vi "Call UI Initialize Device.vi"(8 "error in":errorcluster) -> (0 "error out":errorcluster)   [LabVIEW 2019, in "Initialize.lvlib"]
uses:
  Initialize.lvlib
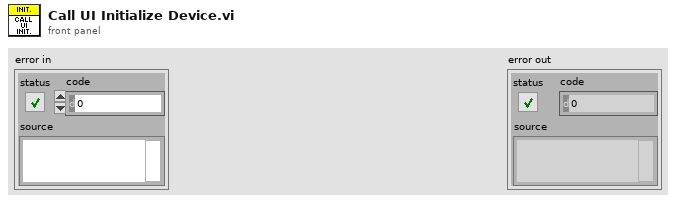
[diagram p1: front panel]
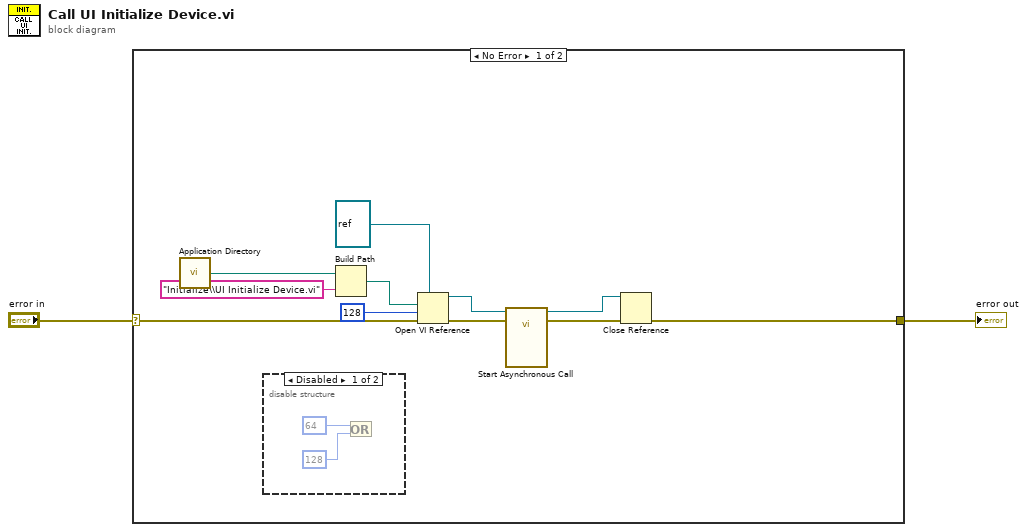
[diagram p0: block diagram]
diagram:
  n1 = case shown="No Error" "error in" {
    selector: "error in" -> [w8 w16]
    tunnel: [w3 w16] -> w1
    frame No Error {
      n2 = call <vilib>:"Application Directory.vi"() -> ("Application Directory"=w10:path)
      n3 = disable-structure shown="Disabled" {
        frame Disabled {
          n4 = Or(x=64 ("options"), y=128 ("options")) -> ()  [unwired: 1 out]
        }
        frame Enabled {
        }
      }
      n5 = Build Path(base path=w10, name or relative path="Initialize\\UI Initialize Device.vi") -> (appended path=w7:path)
      n6 = Open VI Reference(type specifier VI Refnum (for type only)=refnum<vi> refnum, vi path=w7, options=128, error in (no error)=w8) -> (vi reference=w13:refnum<vi>, error out=w12:errorcluster)  [unwired: 2 in]
      n7 = call-by-ref "Start Asynchronous Call"(reference=w13, error in=w12) -> (reference out=w4:refnum<vi>, error out=w5:errorcluster)  [unwired: 11 in, 1 out]
      n8 = Close Reference(reference=w4, error in (no error)=w5) -> (error out=w3:errorcluster)
    }
    frame Error {
    }
  }
  "error out" <- w1
